vi "Get Analog Outputs.vi"(8 "error in (no error)":errorcluster, 11 "GripsMaster in":refnum<class "GripsMaster.lvclass">) -> (0 "error out":errorcluster, 2 "Analog Values":T1, 3 "GripsMaster out":refnum<class "GripsMaster.lvclass">)   [LabVIEW 2013, in "GripsMaster.lvclass"]
uses:
  GripsMaster.lvclass
  controls/Analog Values.ctl
  GripsMaster.lvclass/GripsMaster.ctl
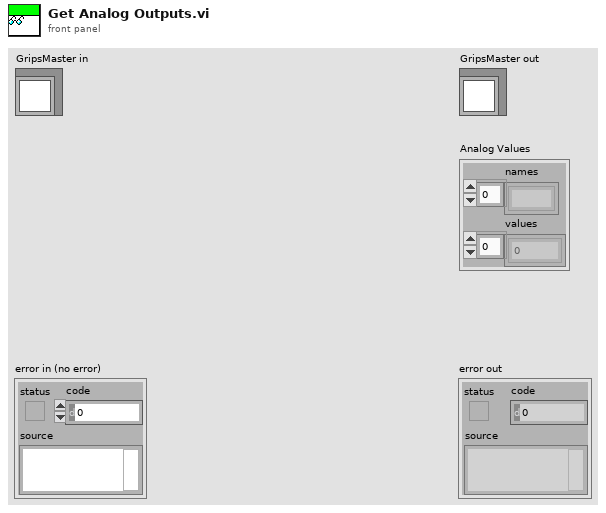
[diagram p1: front panel]
types:
  T1 = typedef "Analog Values.ctl" = cluster{"names":string[], "values":dbl[]}
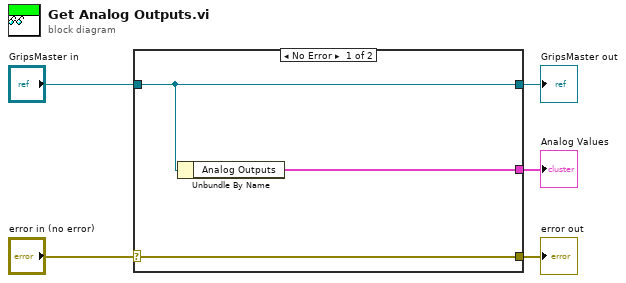
[diagram p0: block diagram]
diagram:
  n1 = case shown="No Error" "error in (no error)" {
    selector: "error in (no error)" -> [w8 w9]
    tunnel: [w8 w9] -> w4
    tunnel: [w7 w10] -> w2
    tunnel: "GripsMaster in" -> [w7 w10]
    tunnel: [w6 _] -> w1
    frame No Error {
      n2 = Unbundle By Name(w7) -> ("Analog Outputs"=w6:T1)
    }
    frame Error {
    }
  }
  "error out" <- w4
  "GripsMaster out" <- w2
  "Analog Values" <- w1
